vi "Test Parameters.vi"(11 "Test Case In":refnum<class "Param Unit Test.lvclass">) -> (0 "error out":errorcluster, 3 "Test Case Out":refnum<class "Param Unit Test.lvclass">)   [LabVIEW 2019, in "Param Unit Test.lvclass"]
uses:
  Param Unit Test.lvclass
  C:/Program Files (x86)/National Instruments/LabVIEW 2024/vi.lib/Astemes/LUnit/Test Case.lvclass
  Param Unit Test.lvclass/Param Unit Test.ctl
  <vilib>/Astemes/LUnit/Test Case.lvclass/Test Case.ctl
  4993e8ee-a06a-463a-9684-69129f64d5ce.vi
  <vilib>/Astemes/LUnit/Core/LUnit Test Case/Private/Append Pass Result.vi
  <vilib>/Astemes/LUnit/Core/LUnit Test Case/Private/Append Fail Result.vi
  4993e8ee-a06a-463a-9684-69129f64d5ce.vi/9c5d11cd-9439-4240-a1ee-d9baace9c924.vi
  <vilib>/Astemes/LUnit/Core/LUnit Test Case/Private/Run In UI.vi
  <vilib>/Utility/error.llb/Clear Errors.vi
  Libraries/Inversor/Inversor.lvlib
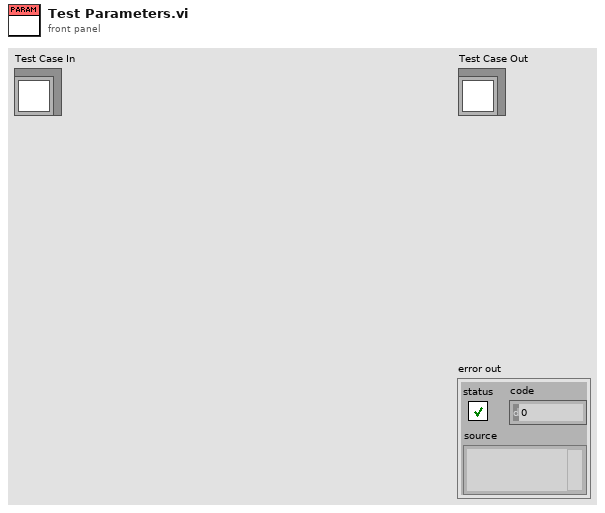
[diagram p1: front panel]
types:
  T1 = enum16{"Set Voltage", "Set Frecuency", "Set Speed", "Set Current"}
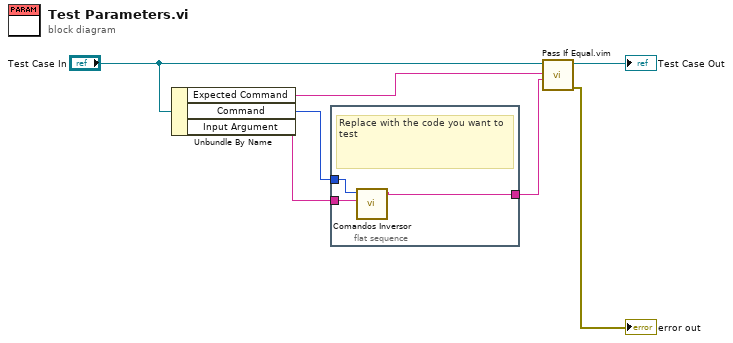
[diagram p0: block diagram]
diagram:
  n1 = Unbundle By Name("Test Case In") -> ("Expected Command"=w3:string, "Command"=w4:T1, "Input Argument"=w1:string)
  n2 = flat-sequence {
    tunnel: w4 -> [w10]
    tunnel: [w8] -> w2
    tunnel: w1 -> [w9]
    frame #0 {
      # "Replace with the code you want to test"
      n3 = call "Comandos Inversor.vi"("Argument"=w9, "Command"=w10) -> ("Command"=w8:string)  [unwired: 9 in]
    }
  }
  n4 = call "Pass If Equal.vim"("Actual"=w2, "Expected"=w3, "LUnit Test Case In"="Test Case In") -> ("error out"=→"error out":errorcluster, "LUnit Test Case Out"=→"Test Case Out":refnum<class "Param Unit Test.lvclass">)  [unwired: 7 in]
